vi "lithographystart.vi"() -> ()   [LabVIEW 2016]
uses:
  Controls/lithography_Control.ctl
panel:
  in  "Ordered Litho data":T1(array[cluster])
  in  "Nanosurf_Easyscan_2.IProxyScan":refnum<k7>
  in  "error in (no error) 2":errorcluster
  in  "Nanosurf_Easyscan_2.IProxyLitho 2":refnum<k7>
  in  "Application":refnum<k7>
  in  "Scan":refnum<k7>
  out "error out":errorcluster
  in  "error in (no error)":errorcluster
  in  "Ordered Lithography Data":T1(array[cluster])
  in  "Litho":refnum<k7>
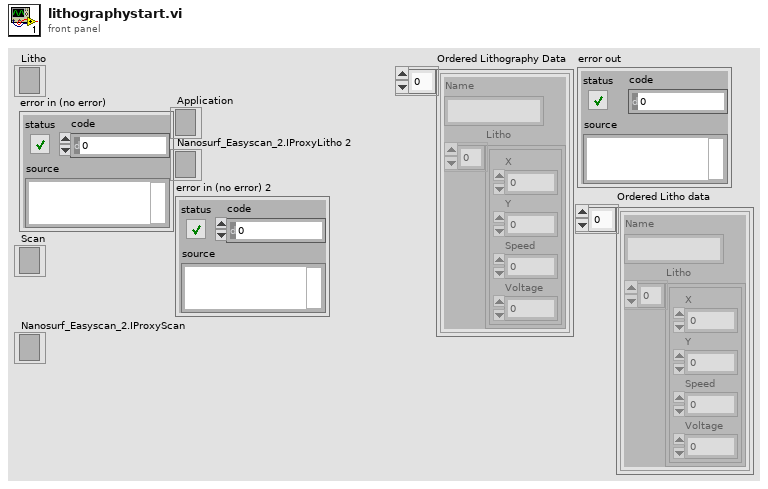
[diagram p1: front panel]
types:
  T1 = cluster{"Name":string, "Litho":cluster{"X":dbl, "Y":dbl, "Speed":dbl, "Voltage":dbl}[]}[]
  T2 = typedef "lithography_Control.ctl" = enum16{"open", "set_param", "litho", "translate", "close", "init"}
  T3 = cluster{"Scan":refnum<k7>, "Litho":refnum<k7>, "Application":refnum<k7>}
  T4 = cluster{"X":dbl, "Y":dbl, "Speed":dbl, "Voltage":dbl}[]
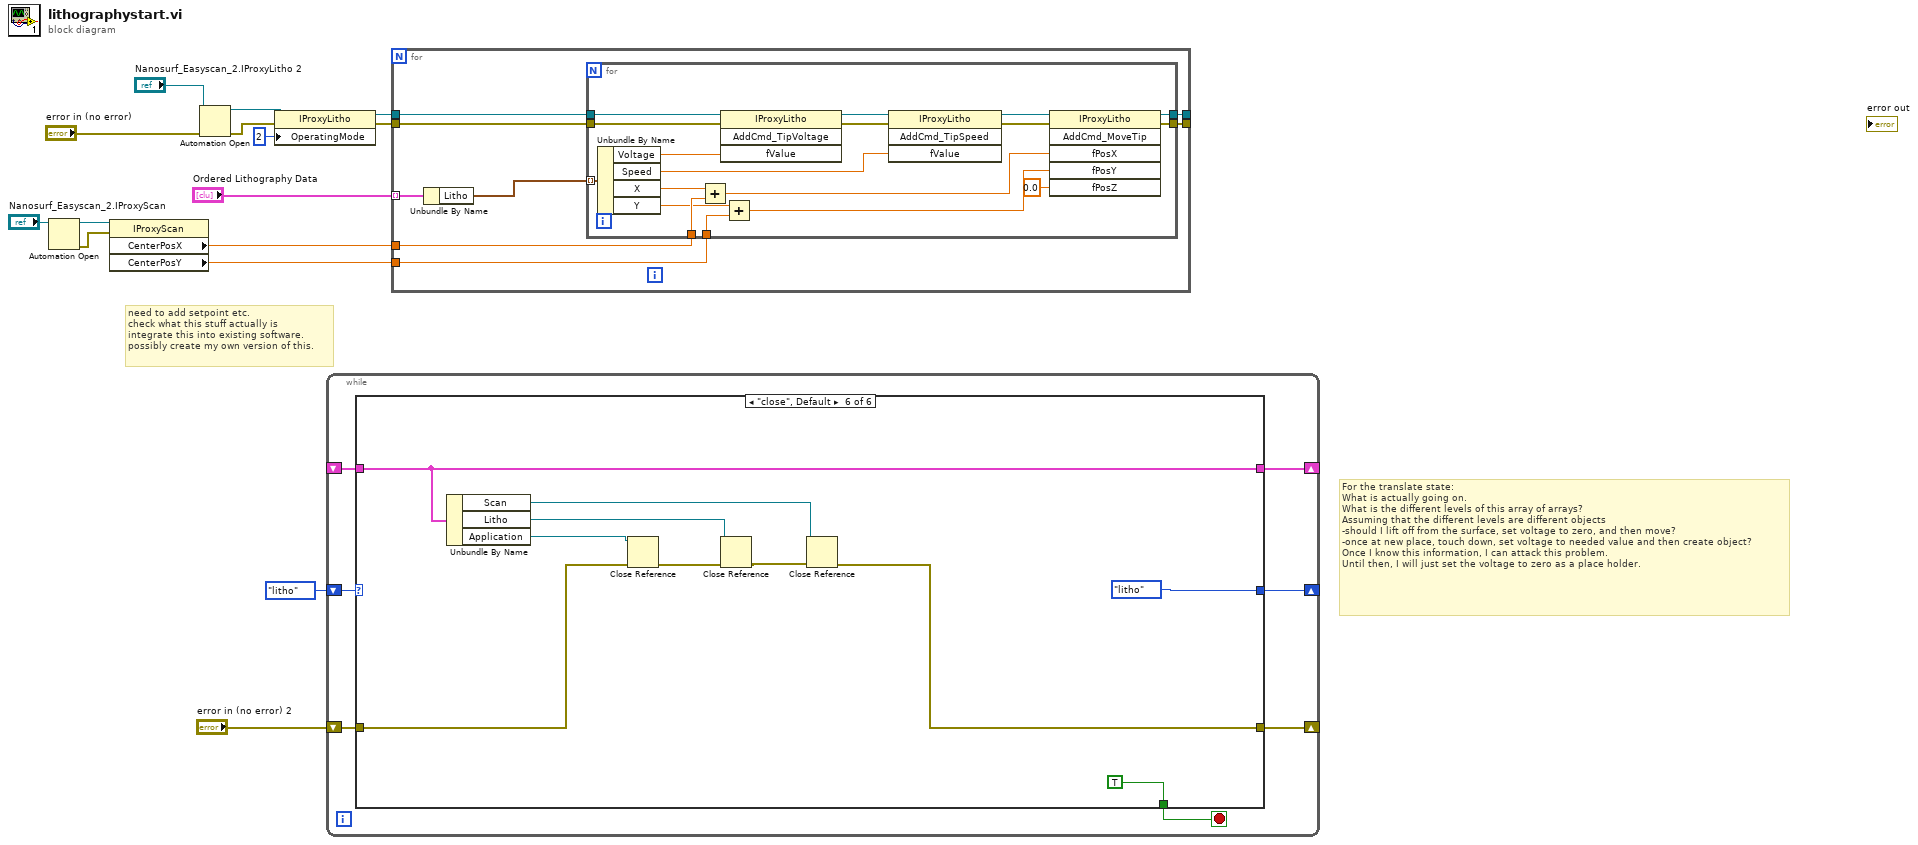
[diagram p0: block diagram]
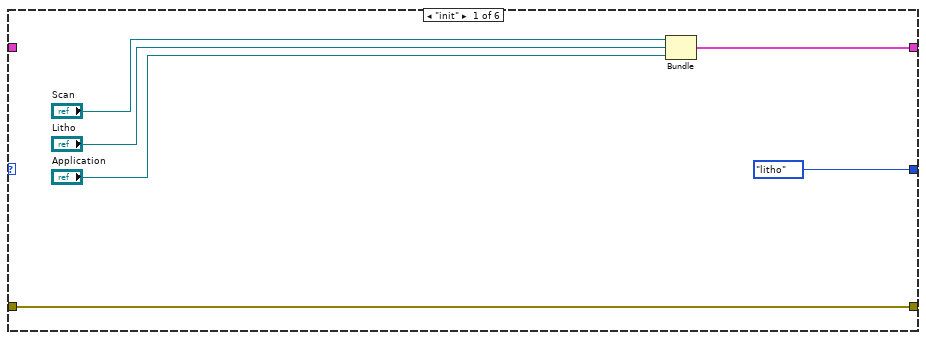
[diagram p2: hidden frame]
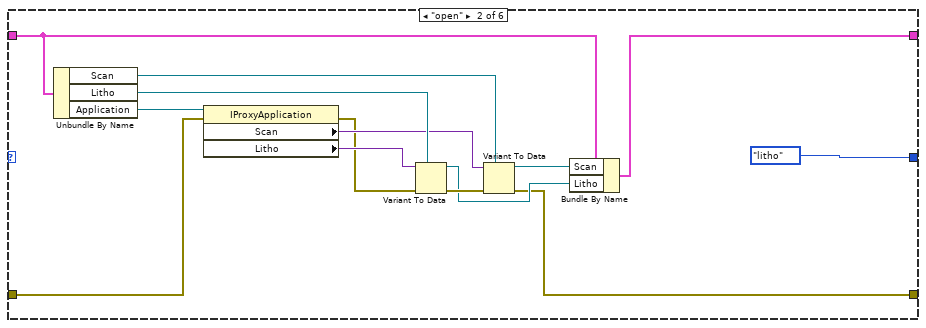
[diagram p3: hidden frame]
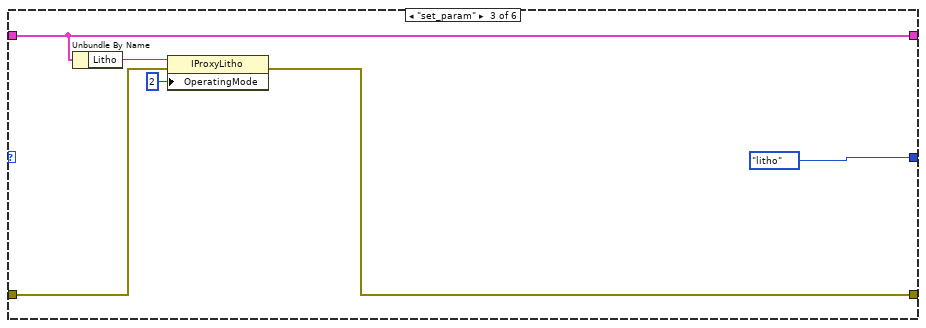
[diagram p4: hidden frame]
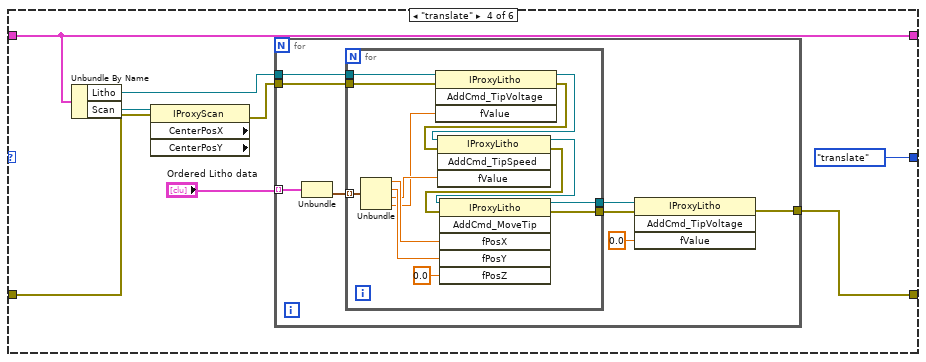
[diagram p5: hidden frame]
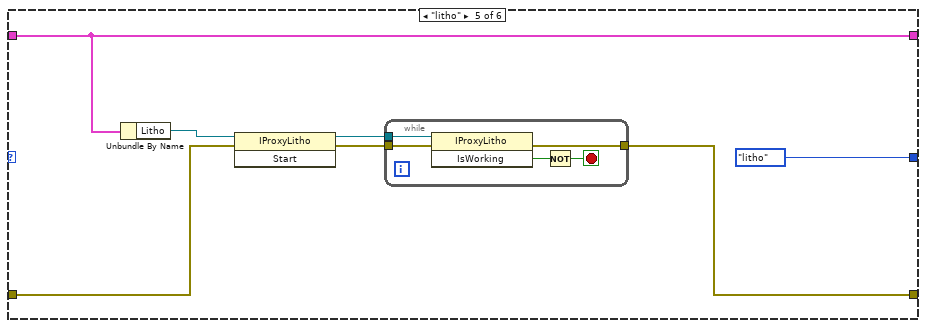
[diagram p6: hidden frame]
diagram:
  # "For the translate state:\nWhat is actually going on. \nWhat is the different levels of this array of arrays?\nAssuming that the different levels are different objects\n-should I lift off from the surface, set voltage to zero, and then move?\n-once at new place, touch down, set voltage to needed value and then create object?\nOnce I know this information, I can attack this problem.\nUntil then, I will just set the voltage to zero as a place holder."
  # "need to add setpoint etc.\ncheck what this stuff actually is\nintegrate this into existing software.\npossibly create my own version of this."
  n1 = Automation Open(Automation Refnum="Nanosurf_Easyscan_2.IProxyScan") -> (Automation Refnum=w8:refnum<k7>, error out=w7:errorcluster)  [unwired: 3 in]
  n2 = property class="IProxyScan"(reference=w8, error in=w7) -> ("CenterPosX"=w6:dbl, "CenterPosY"=w5:dbl)  [unwired: 2 out]
  n3 = Automation Open(error in (no error)="error in (no error)", Automation Refnum="Nanosurf_Easyscan_2.IProxyLitho 2") -> (Automation Refnum=w15:refnum<k7>, error out=w11:errorcluster)  [unwired: 2 in]
  n4 = property class="IProxyLitho"(reference=w15, error in=w11, "OperatingMode"=2) -> (reference out=w13:refnum<k7>, error out=w12:errorcluster)
  n5 = while {
    shift-right: [w21] -> _
    shift-left: lithography_Control."litho" -> [w22]
    shift-right: [w20] -> _
    shift-left: _ -> [w19]
    shift-right: [w17] -> _
    shift-left: "error in (no error) 2" -> [w18]
    stop <- w16 stop-if-true
    n6 = case shown="\"close\", Default" w22 {
      tunnel: [lithography_Control."litho" lithography_Control."litho" lithography_Control."litho" lithography_Control."translate" lithography_Control."litho" lithography_Control."litho"] -> w21
      tunnel: [w24 w39 w47 w55 w82 w98] -> w20
      tunnel: w19 -> [_ w40 w47 w55 w82 w98]
      tunnel: w18 -> [w23 w37 w45 w51 w80 w92]
      tunnel: [w23 w29 w44 w49 w79 w91] -> w17
      tunnel: [_ _ _ _ _ TRUE] -> w16
      frame "init" {
        n7 = Bundle("Scan"="Scan", "Litho"="Litho", "Application"="Application") -> (w24:T3)  [unwired: 1 in]
      }
      frame "open" {
        n8 = Unbundle By Name(w40) -> ("Scan"=w36:refnum<k7>, "Litho"=w35:refnum<k7>, "Application"=w41:refnum<k7>)
        n9 = property class="IProxyApplication"(reference=w41, error in=w37) -> (error out=w30:errorcluster, "Scan"=w34:variant, "Litho"=w33:variant)  [unwired: 1 out]
        n10 = Variant To Data(error in=w30, type=w35, Variant=w33) -> (data=w31:refnum<k7>, error out=w38:errorcluster)
        n11 = Variant To Data(error in=w38, type=w36, Variant=w34) -> (data=w32:refnum<k7>, error out=w29:errorcluster)
        n12 = Bundle By Name(cluster=w40, "Scan"=w32, "Litho"=w31) -> (w39:T3)
      }
      frame "set_param" {
        n13 = Unbundle By Name(w47) -> ("Litho"=w46:refnum<k7>)
        n14 = property class="IProxyLitho"(reference=w46, error in=w45, "OperatingMode"=2) -> (error out=w44:errorcluster)  [unwired: 1 out]
      }
      frame "translate" {
        n15 = Unbundle By Name(w55) -> ("Litho"=w53:refnum<k7>, "Scan"=w54:refnum<k7>)
        n16 = property class="IProxyScan" props=["CenterPosX", "CenterPosY"](reference=w54, error in=w51) -> (error out=w52:errorcluster)  [unwired: 3 out]
        n17 = for {
          tunnel: w53 -> [w64]
          tunnel: w52 -> [w63]
          tunnel: "Ordered Litho data" -> [w62] mode=indexing
          tunnel: [w57] -> w49
          n18 = Unbundle(w62) -> ("Litho"=w61:T4)  [unwired: 1 out]
          n19 = for {
            tunnel: w64 -> [w78]
            tunnel: w63 -> [w77]
            tunnel: w61 -> [w72] mode=indexing
            tunnel: [w67] -> w60
            tunnel: [w65] -> w58
            n20 = Unbundle(w72) -> ("X"=w71:dbl, "Y"=w70:dbl, "Speed"=w69:dbl, "Voltage"=w68:dbl)
            n21 = invoke class="IProxyLitho" method="AddCmd_TipVoltage"(reference=w78, error in=w77, "fValue"=w68) -> (reference out=w75:refnum<k7>, error out=w76:errorcluster)  [unwired: 1 in, 2 out]
            n22 = invoke class="IProxyLitho" method="AddCmd_TipSpeed"(reference=w75, error in=w76, "fValue"=w69) -> (reference out=w74:refnum<k7>, error out=w73:errorcluster)  [unwired: 1 in, 2 out]
            n23 = invoke class="IProxyLitho" method="AddCmd_MoveTip"(reference=w74, error in=w73, "fPosX"=w71, "fPosY"=w70, "fPosZ"=0.0) -> (reference out=w67:refnum<k7>, error out=w65:errorcluster)  [unwired: 1 in, 4 out]
          }
          n24 = invoke class="IProxyLitho" method="AddCmd_TipVoltage"(reference=w60, error in=w58, "fValue"=0.0) -> (error out=w57:errorcluster)  [unwired: 1 in, 3 out]
        }
      }
      frame "litho" {
        n25 = Unbundle By Name(w82) -> ("Litho"=w81:refnum<k7>)
        n26 = invoke class="IProxyLitho" method="Start"(reference=w81, error in=w80) -> (reference out=w83:refnum<k7>, error out=w84:errorcluster)  [unwired: 1 in, 1 out]
        n27 = while {
          tunnel: w83 -> [w90]
          tunnel: w84 -> [w89]
          tunnel: [w88] -> w79
          stop <- w86 stop-if-true
          n28 = invoke class="IProxyLitho" method="IsWorking"(reference=w90, error in=w89) -> (error out=w88:errorcluster, "IsWorking"=w87:bool)  [unwired: 1 in, 1 out]
          n29 = Not(x=w87) -> (.not. x?=w86:bool)
        }
      }
      frame "close", Default {
        n30 = Unbundle By Name(w98) -> ("Scan"=w95:refnum<k7>, "Litho"=w96:refnum<k7>, "Application"=w97:refnum<k7>)
        n31 = Close Reference(reference=w97, error in (no error)=w92) -> (error out=w94:errorcluster)
        n32 = Close Reference(reference=w96, error in (no error)=w94) -> (error out=w93:errorcluster)
        n33 = Close Reference(reference=w95, error in (no error)=w93) -> (error out=w91:errorcluster)
      }
    }
  }
  n34 = for {
    tunnel: w13 -> [w108]
    tunnel: w12 -> [w107]
    tunnel: [w106] -> _
    tunnel: [w105] -> _
    tunnel: "Ordered Lithography Data" -> [w104] mode=indexing
    tunnel: w6 -> [w102]
    tunnel: w5 -> [w101]
    n35 = Unbundle By Name(w104) -> ("Litho"=w103:T4)
    n36 = for {
      tunnel: w107 -> [w125]
      tunnel: [w119] -> w105
      tunnel: w108 -> [w126]
      tunnel: [w120] -> w106
      tunnel: w103 -> [w118] mode=indexing
      tunnel: w102 -> [w113]
      tunnel: w101 -> [w111]
      n37 = Unbundle By Name(w118) -> ("Voltage"=w117:dbl, "Speed"=w116:dbl, "X"=w114:dbl, "Y"=w110:dbl)
      n38 = Add(x=w114, y=w113) -> (x+y=w112:dbl)
      n39 = invoke class="IProxyLitho" method="AddCmd_TipVoltage"(reference=w126, error in=w125, "fValue"=w117) -> (reference out=w124:refnum<k7>, error out=w123:errorcluster)  [unwired: 1 in, 2 out]
      n40 = Add(x=w110, y=w111) -> (x+y=w109:dbl)
      n41 = invoke class="IProxyLitho" method="AddCmd_TipSpeed"(reference=w124, error in=w123, "fValue"=w116) -> (reference out=w122:refnum<k7>, error out=w121:errorcluster)  [unwired: 1 in, 2 out]
      n42 = invoke class="IProxyLitho" method="AddCmd_MoveTip"(reference=w122, error in=w121, "fPosX"=w112, "fPosY"=w109, "fPosZ"=0.0) -> (reference out=w120:refnum<k7>, error out=w119:errorcluster)  [unwired: 1 in, 4 out]
    }
  }
